vi "Scale Ort Data Quad.vi"(10 "Pitch (Arg 2)":string, 11 "Roll (Arg 3)":string) -> (2 "theta_y":dbl, 3 "theta_x":dbl)   [LabVIEW 2014]
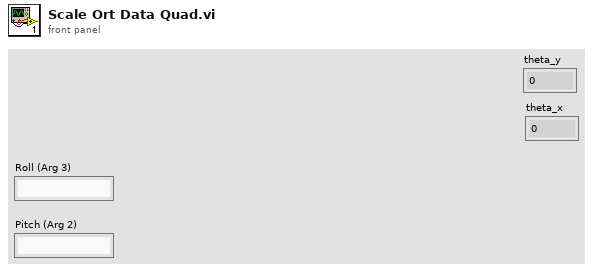
[diagram p1: front panel]
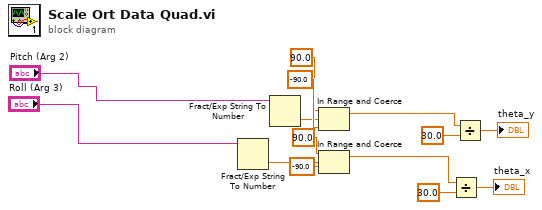
[diagram p0: block diagram]
diagram:
  n1 = Fract/Exp String To Number(string="Roll (Arg 3)") -> (number=w9:dbl)  [unwired: 3 in, 1 out]
  n2 = Fract/Exp String To Number(string="Pitch (Arg 2)") -> (number=w7:dbl)  [unwired: 3 in, 1 out]
  n3 = In Range and Coerce(upper limit=90.0, x=w7, lower limit=-90.0) -> (coerced(x)=w6:dbl)  [unwired: 1 out]
  n4 = In Range and Coerce(upper limit=90.0, x=w9, lower limit=-90.0) -> (coerced(x)=w3:dbl)  [unwired: 1 out]
  n5 = Divide(x=w3, y=30.0) -> (x/y=→"theta_x":dbl)
  n6 = Divide(x=w6, y=30.0) -> (x/y=→"theta_y":dbl)
